vi "PID参数调节.vi"() -> ()   [LabVIEW 2013]
panel:
  in  "比例":dbl=0.43
  in  "积分":dbl=0.12
  in  "微分":dbl=0.23
  in  "目标值":dbl=5.0
  out "过程输出值":dbl format="%_12g"
  out "Waveform Chart":dbl(graph)
  in  "循环时间":dbl=50.0 format="%#_3g"
  in  "初始输入值":dbl
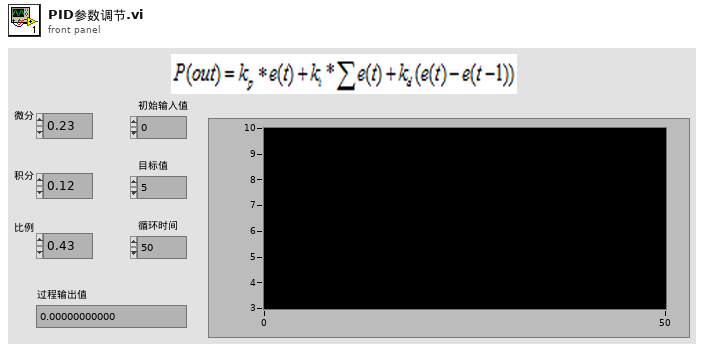
[diagram p1: front panel]
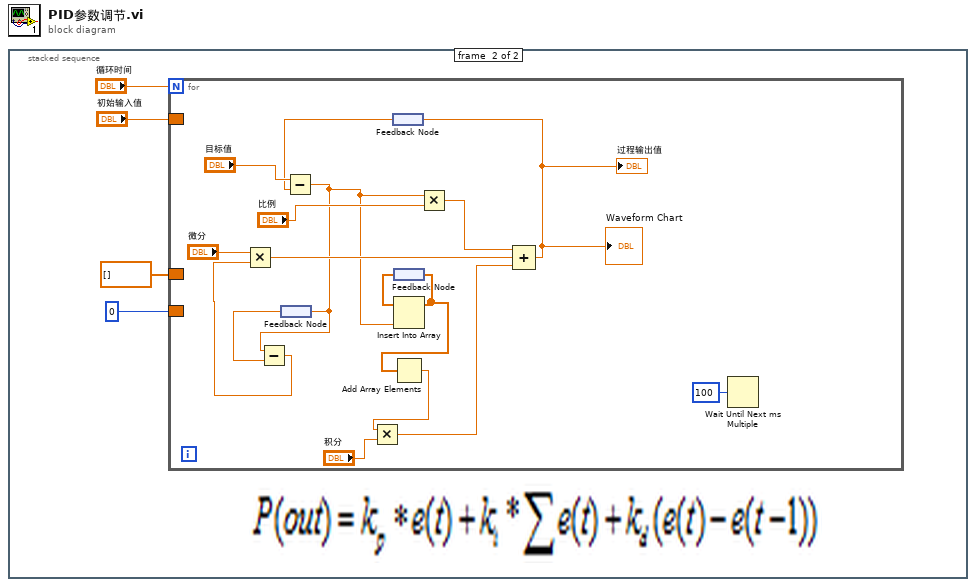
[diagram p0: block diagram]
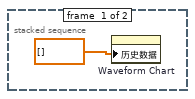
[diagram p2: hidden frame]
diagram:
  n1 = stacked-sequence {
    frame #0 {
      n2 = property on="Waveform Chart" class="WFChart (严格)"("历史数据"=dbl[] [] ("History Data")) -> ()  [unwired: 2 in, 2 out]
    }
    frame #1 {
      n3 = for {
        N: "循环时间" -> [_]
        border: "初始输入值" -> [_]
        border: 0 -> [_]
        border: dbl[] [] -> [_]
        n4 = feedback #1() -> (w8:dbl)
        n5 = feedback #2() -> (w13:dbl)
        n6 = Subtract(x="目标值", y=w13) -> (x-y=w7:dbl)
        n7 = Subtract(x=w7, y=w8) -> (x-y=w6:dbl)
        n8 = Multiply(x="微分", y=w6) -> (x*y=w17:dbl)
        n9 = feedback-in #1(w7) -> ()
        n10 = feedback #3() -> (w11:dbl[])
        n11 = Insert Into Array(array=w11, new element=w7) -> (w10:dbl[])  [unwired: 1 in]
        n12 = feedback-in #3(w10) -> ()
        n13 = Add Array Elements(numeric array=w10) -> (sum=w9:dbl)
        n14 = Multiply(x=w9, y="积分") -> (x*y=w12:dbl)
        n15 = Multiply(x=w7, y="比例") -> (x*y=w16:dbl)
        n16 = Compound Arithmetic op=ADD(w16, w17, w12) -> (w14:dbl)
        "过程输出值" <- w14
        "Waveform Chart" <- w14
        n17 = feedback-in #2(w14) -> ()
        n18 = Wait Until Next ms Multiple(millisecond multiple=u32 100) -> ()  [unwired: 1 out]
      }
    }
  }
